vi "rszvl Get OPC Timeout.vi"(8 "error in (no error)":errorcluster, 11 "VISA resource name":refnum<visa-resource-name>) -> (0 "error out":errorcluster, 2 "OPC Timeout":i32, 3 "VISA resource name out":refnum<visa-resource-name>)   [LabVIEW 2014]
doc: "This VI returns the current value of the driver's OPC timeout in milliseconds. OPC timeout is different from the VISA timeout and it is used by the driver for long-lasting operations, e.g. instrument's acquisition."
uses:
  rszvl_rsidr_core.lvlib
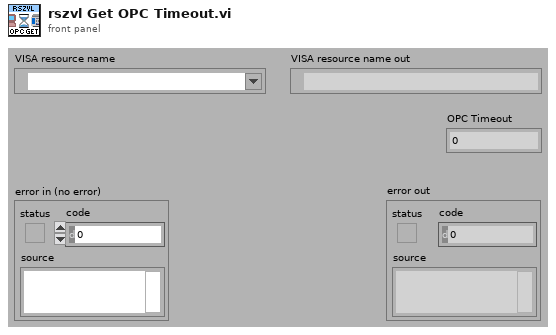
[diagram p1: front panel]
types:
  T1 = typedef "rszvl_rsidr_core.lvlib/type_Session_Data.ctl" = cluster{"Instr type":string, "Instr type for err. msg.":string, "Installed Options":string[], "OPC Timeout":i32, "Query Instrument Status":bool, "Check Range":bool, "Check Options":bool, "Add LF to Write":bool, "Simulate":bool, "Logging":bool, "Logging params":variant, "Interface Type":enum16{"Unknown", "GPIB", "VXI", "GPIB_VXI", "ASRL", "PXI", "TCPIP", "USB", "SOCKET"}, "Fast Sweep":i32, "AdditionalFlags":i32, "WaitBeforeWrite":i32, "WaitBeforeRead":i32, "BinDataChunkSize":i64}
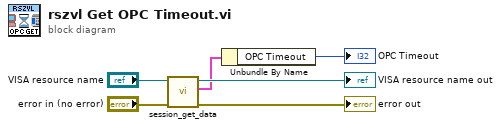
[diagram p0: block diagram]
diagram:
  n1 = call "session_get_data.vi"("error in"="error in (no error)", "VISA resource name"="VISA resource name") -> ("error out"=→"error out":errorcluster, "Session User Data out"=w1:T1, "VISA resource name out"=→"VISA resource name out":refnum<visa-resource-name>)  [unwired: 7 in]
  n2 = Unbundle By Name(w1) -> ("OPC Timeout"=→"OPC Timeout":i32)
